vi "Determine Package Type.vi"(7 "Die_Coordinates":string[](array[string]), 8 "error in (no error)":errorcluster, 10 "Die_X_Y":string, 11 "USID":T1 max=15) -> (0 "error out":errorcluster, 3 "Package_Type":string)   [LabVIEW 2013]
uses:
  Controls/USID.ctl
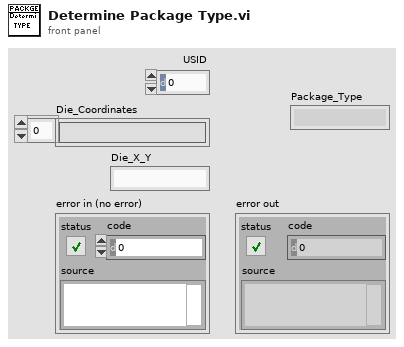
[diagram p1: front panel]
types:
  T1 = typedef "USID.ctl" = u8
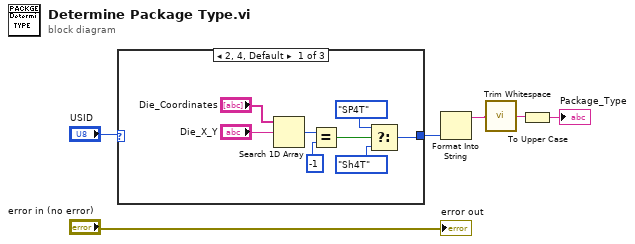
[diagram p0: block diagram]
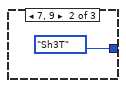
[diagram p2: hidden frame]
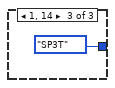
[diagram p3: hidden frame]
diagram:
  n1 = case shown="2, 4, Default" "USID" {
    tunnel: [w7 enum16{"SP4T", "SP3T", "Sh3T", "Sh4T"}."Sh3T" ("Die Type 2") enum16{"SP4T", "SP3T", "Sh3T", "Sh4T"}."SP3T" ("Die Type 2")] -> w5
    frame 2, 4, Default {
      n2 = Search 1D Array(1D array="Die_Coordinates", element="Die_X_Y") -> (index of element=w10:i32)  [unwired: 1 in]
      n3 = Equal?(x=w10, y=-1) -> (x = y?=w12:bool)
      n4 = Select(t=enum16{"SP4T", "SP3T", "Sh3T", "Sh4T"}."SP4T" ("Die Type 2"), s=w12, f=enum16{"SP4T", "SP3T", "Sh3T", "Sh4T"}."Sh4T" ("Die Type 2")) -> (s? t:f=w7:enum16{"SP4T", "SP3T", "Sh3T", "Sh4T"})
    }
    frame 7, 9 {
    }
    frame 1, 14 {
    }
  }
  n5 = Format Into String(w5) -> (resulting string=w4:string)  [unwired: 3 in, 1 out]
  n6 = call <vilib>:"Trim Whitespace.vi"("string"=w4) -> ("trimmed string"=w3:string)  [unwired: 1 in]
  n7 = To Upper Case(1:w3) -> (0:→"Package_Type":string)
  "error out" <- "error in (no error)"
